vi "XMTmotorSample.vi"() -> ()   [LabVIEW 2018]
uses:
  DLL/XMT_DLL_SER.dll
panel:
  in  "COM":u64=3
  in  "运行停止":bool
  in  "计数清零":bool
  in  "低分辨率":bool
  in  "高分辨率":bool
  in  "MoveX_f 4":dbl=10.0
  in  "设置运行速度":bool
  out "RData 6":sgl
  out "int":i8
  in  "枚举":enum16{"开环O 79", "闭环C 67"}(ring)
  out "返回类型":u8
  out "ReData":u8
  in  "读取下位机单位":bool
  out "数值":i32
  in  "设置下位机单位":bool
  in  "文本下拉列表":u16(ring) items=["0角秒; ", "1毫弧度; ", "2微弧度; ", "3度; ", "4光栅尺一刻度;"]
  out "RData 5":u8
  in  "读取开闭环":bool
  in  "设置开闭环":bool
  in  "读取最大速度":bool
  in  "tmpflagRe":u8=1
  out "RData 4":sgl
  in  "读取位置信息":bool
  in  "MoveX_f 3":dbl
  in  "设置速度":bool
  in  "JOrXFlag":u8
  out "RData 3":sgl
  in  "ReFlag 3":u8
  in  "返回零位置":bool
  out "RData 2":sgl
  in  "ReFlag 2":u8
  in  "MoveX_f 2":dbl=10.0
  in  "位移增量":bool
  out "错误输出":errorcluster
  in  "停止":bool
  out "RData":sgl
  in  "Address":u8=1
  in  "Ch":u8
  in  "ReFlag":u8
  in  "MoveX_f":dbl=24.0
  in  "绝对位置":bool
  # "开环O:79"
  # "闭环C:67"
  # "0角秒 1毫弧度  2微弧度 3度 4光栅尺一刻度"
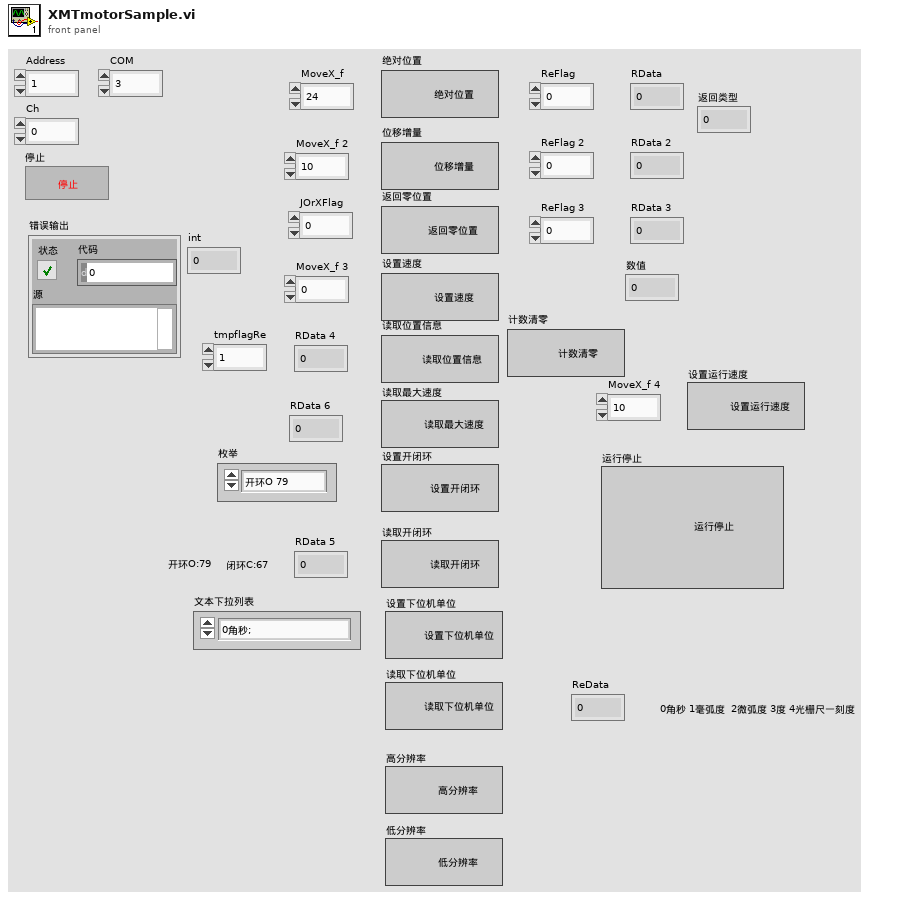
[diagram p1: front panel]
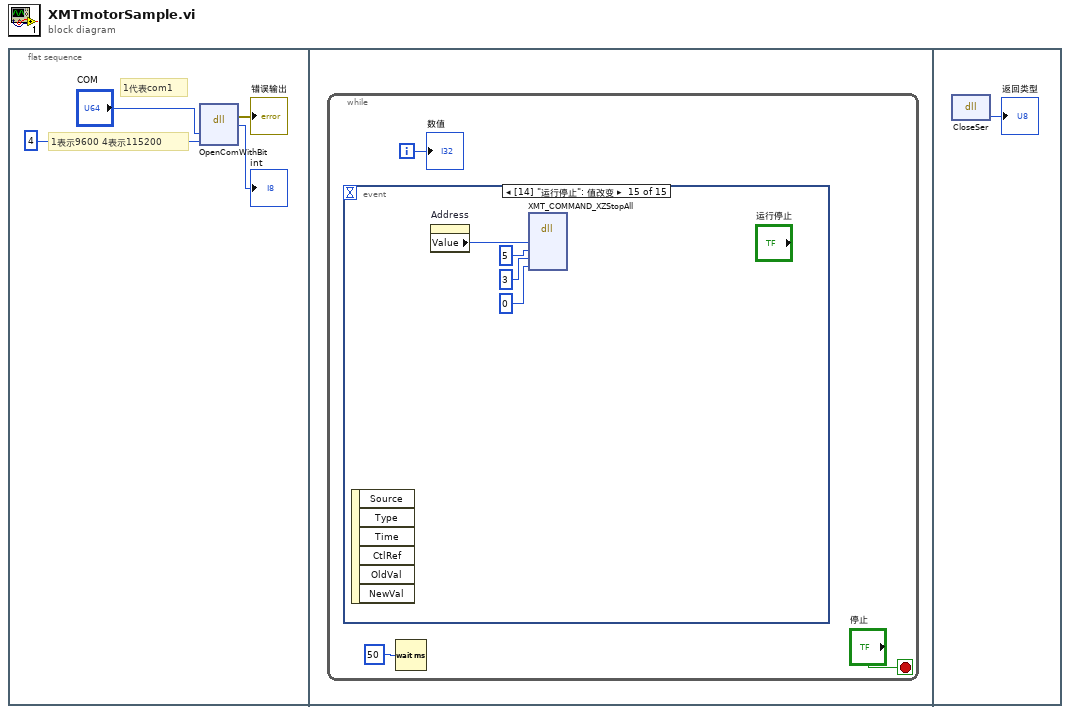
[diagram p0: block diagram]
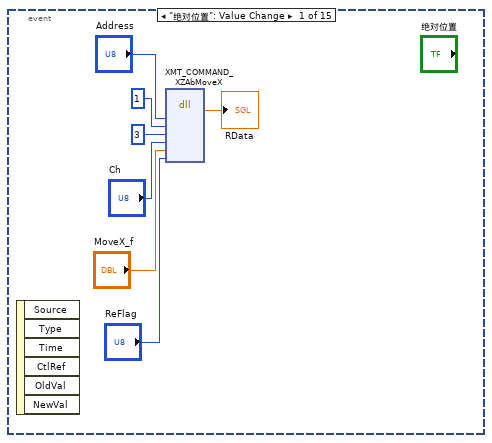
[diagram p2: hidden frame]
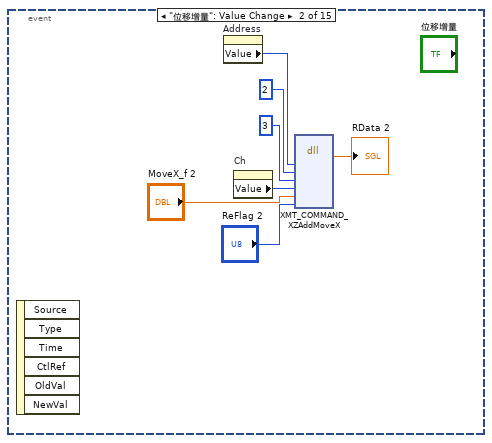
[diagram p3: hidden frame]
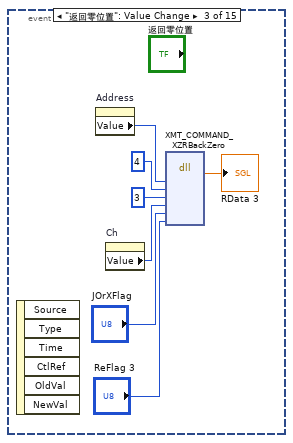
[diagram p4: hidden frame]
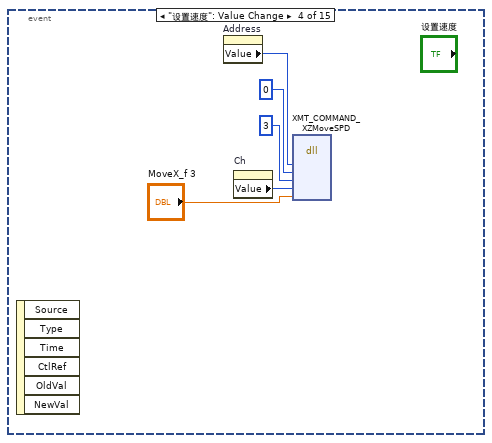
[diagram p5: hidden frame]
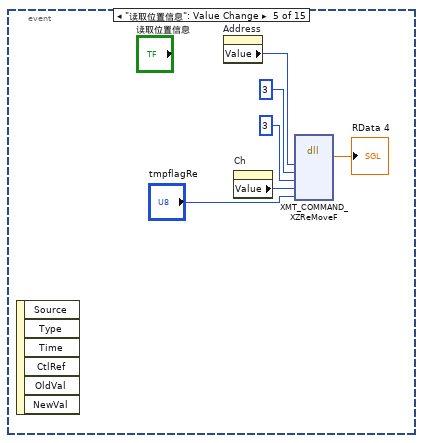
[diagram p6: hidden frame]
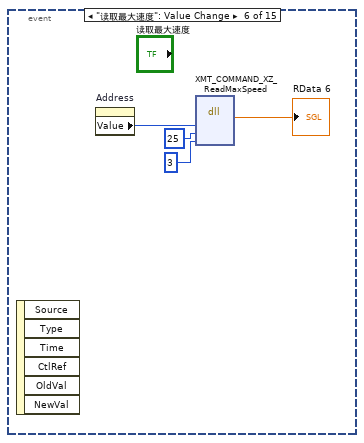
[diagram p7: hidden frame]
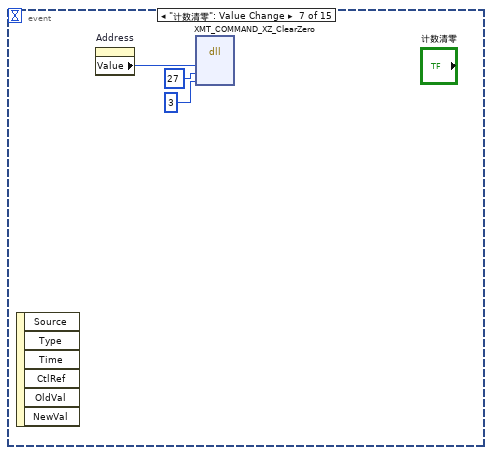
[diagram p8: hidden frame]
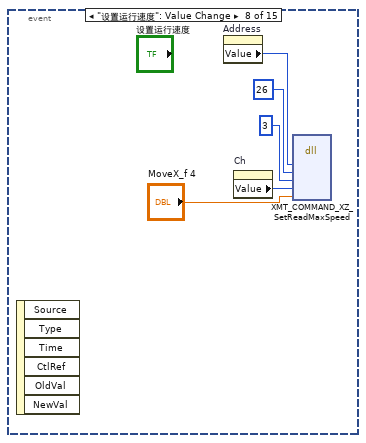
[diagram p9: hidden frame]
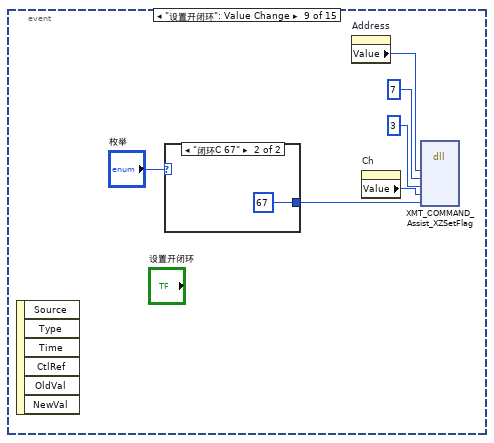
[diagram p10: hidden frame]
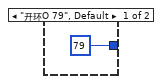
[diagram p11: hidden frame]
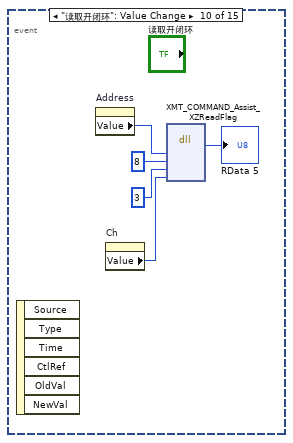
[diagram p12: hidden frame]
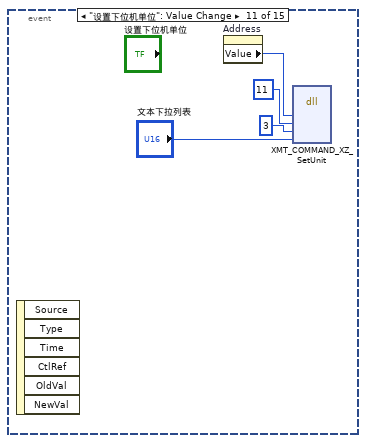
[diagram p13: hidden frame]
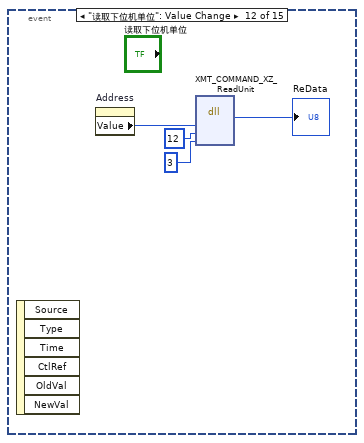
[diagram p14: hidden frame]
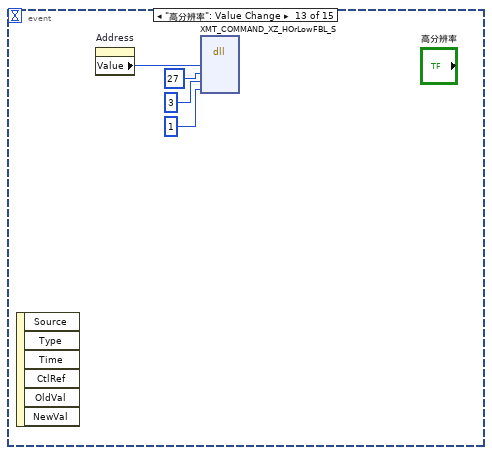
[diagram p15: hidden frame]
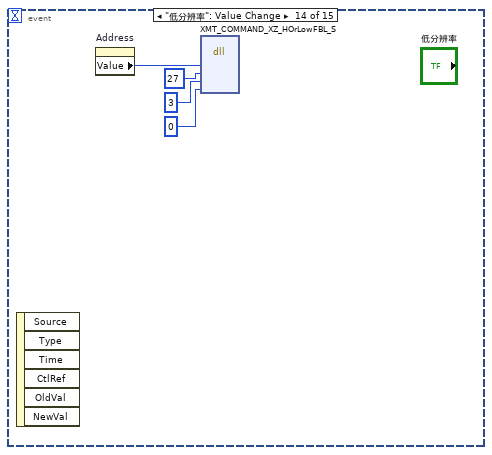
[diagram p16: hidden frame]
diagram:
  n1 = flat-sequence {
    frame #0 {
      # "1表示9600 4表示115200"
      # "1代表com1"
      n2 = dll-call lib="C:/Users/cy3486/OneDrive/Desktop/OPO_control_scripts/SHG_motor_control/DLL/XMT_DLL_SER.dll" fn="OpenComWithBit"("m_com"="COM", "BaudRate"=u8 4) -> (error out=→"错误输出":errorcluster, "int"=→"int":i8)  [unwired: 5 in, 1 out]
    }
    frame #1 {
      n3 = while {
        i -> [w5]
        stop <- "停止" stop-if-true
        n4 = event shown="[14] \"运行停止\": 值改变" {
          selector: _ -> [_ _ _ _ _ _ _ _ _ _ _ _ _ _ _]
          dyn-events: _ -> [_ _ _ _ _ _ _ _ _ _ _ _ _ _ _]
          timeout: _ -> [_ _ _ _ _ _ _ _ _ _ _ _ _ _ _]
          event "绝对位置": Value Change {
            n5 = event-data() -> ()  [unwired: 1 in, 6 out]
            n6 = dll-call lib="C:/Users/cy3486/OneDrive/Desktop/OPO_control_scripts/SHG_motor_control/DLL/XMT_DLL_SER.dll" fn="XMT_COMMAND_XZAbMoveX"("Address"="Address", "Command_B3"=u16 1, "Command_B4"=u16 3 ("Command_B3"), "Ch"="Ch", "MoveX_f"="MoveX_f", "ReFlag"="ReFlag") -> ("RData"=→"RData":sgl)  [unwired: 9 in, 2 out]
          }
          event "位移增量": Value Change {
            n7 = event-data() -> ()  [unwired: 1 in, 6 out]
            n8 = property on="Address" class="DigNum (严格)"() -> ("Value"=w15:u8)  [unwired: 2 in, 2 out]
            n9 = property on="Ch" class="DigNum (严格)"() -> ("Value"=w16:u8)  [unwired: 2 in, 2 out]
            n10 = dll-call lib="C:/Users/cy3486/OneDrive/Desktop/OPO_control_scripts/SHG_motor_control/DLL/XMT_DLL_SER.dll" fn="XMT_COMMAND_XZAddMoveX"("Address"=w15, "Command_B3"=u16 2, "Command_B4"=u16 3 ("Command_B3"), "Ch"=w16, "MoveX_f"="MoveX_f 2", "ReFlag"="ReFlag 2") -> ("RData"=→"RData 2":sgl)  [unwired: 9 in, 2 out]
          }
          event "返回零位置": Value Change {
            n11 = event-data() -> ()  [unwired: 1 in, 6 out]
            n12 = property on="Address" class="DigNum (严格)"() -> ("Value"=w24:u8)  [unwired: 2 in, 2 out]
            n13 = property on="Ch" class="DigNum (严格)"() -> ("Value"=w23:u8)  [unwired: 2 in, 2 out]
            n14 = dll-call lib="C:/Users/cy3486/OneDrive/Desktop/OPO_control_scripts/SHG_motor_control/DLL/XMT_DLL_SER.dll" fn="XMT_COMMAND_XZRBackZero"("Address"=w24, "Command_B3"=u16 4, "Command_B4"=u16 3 ("Command_B3"), "Ch"=w23, "JOrXFlag"="JOrXFlag", "ReFlag"="ReFlag 3") -> ("RData"=→"RData 3":sgl)  [unwired: 9 in, 2 out]
          }
          event "设置速度": Value Change {
            n15 = event-data() -> ()  [unwired: 1 in, 6 out]
            n16 = property on="Address" class="DigNum (严格)"() -> ("Value"=w30:u8)  [unwired: 2 in, 2 out]
            n17 = property on="Ch" class="DigNum (严格)"() -> ("Value"=w31:u8)  [unwired: 2 in, 2 out]
            n18 = dll-call lib="C:/Users/cy3486/OneDrive/Desktop/OPO_control_scripts/SHG_motor_control/DLL/XMT_DLL_SER.dll" fn="XMT_COMMAND_XZMoveSPD"("Address"=w30, "Command_B3"=u16 0, "Command_B4"=u16 3 ("Command_B3"), "Ch"=w31, "MoveX_f"="MoveX_f 3") -> ()  [unwired: 9 in, 2 out]
          }
          event "读取位置信息": Value Change {
            n19 = event-data() -> ()  [unwired: 1 in, 6 out]
            n20 = property on="Address" class="DigNum (严格)"() -> ("Value"=w35:u8)  [unwired: 2 in, 2 out]
            n21 = property on="Ch" class="DigNum (严格)"() -> ("Value"=w36:u8)  [unwired: 2 in, 2 out]
            n22 = dll-call lib="C:/Users/cy3486/OneDrive/Desktop/OPO_control_scripts/SHG_motor_control/DLL/XMT_DLL_SER.dll" fn="XMT_COMMAND_XZReMoveF"("Address"=w35, "Command_B3"=u16 3, "Command_B4"=u16 3 ("Command_B3"), "Ch"=w36, "tmpflagRe"="tmpflagRe") -> ("RData"=→"RData 4":sgl)  [unwired: 8 in, 2 out]
          }
          event "读取最大速度": Value Change {
            n23 = event-data() -> ()  [unwired: 1 in, 6 out]
            n24 = property on="Address" class="DigNum (严格)"() -> ("Value"=w41:u8)  [unwired: 2 in, 2 out]
            n25 = dll-call lib="C:/Users/cy3486/OneDrive/Desktop/OPO_control_scripts/SHG_motor_control/DLL/XMT_DLL_SER.dll" fn="XMT_COMMAND_XZ_ReadMaxSpeed"("Address"=w41, "Command_B3"=u16 25, "Command_B4"=u16 3 ("Command_B3")) -> ("RData"=→"RData 6":sgl)  [unwired: 6 in, 2 out]
          }
          event "计数清零": Value Change {
            n26 = event-data() -> ()  [unwired: 1 in, 6 out]
            n27 = property on="Address" class="DigNum (严格)"() -> ("Value"=w44:u8)  [unwired: 2 in, 2 out]
            n28 = dll-call lib="C:/Users/cy3486/OneDrive/Desktop/OPO_control_scripts/SHG_motor_control/DLL/XMT_DLL_SER.dll" fn="XMT_COMMAND_XZ_ClearZero"("Address"=w44, "Command_B3"=u16 27, "Command_B4"=u16 3 ("Command_B3")) -> ()  [unwired: 7 in, 2 out]
          }
          event "设置运行速度": Value Change {
            n29 = event-data() -> ()  [unwired: 1 in, 6 out]
            n30 = property on="Address" class="DigNum (严格)"() -> ("Value"=w48:u8)  [unwired: 2 in, 2 out]
            n31 = property on="Ch" class="DigNum (严格)"() -> ("Value"=w49:u8)  [unwired: 2 in, 2 out]
            n32 = dll-call lib="C:/Users/cy3486/OneDrive/Desktop/OPO_control_scripts/SHG_motor_control/DLL/XMT_DLL_SER.dll" fn="XMT_COMMAND_XZ_SetReadMaxSpeed"("Address"=w48, "Command_B3"=u16 26, "Command_B4"=u16 3 ("Command_B3"), "Ch"=w49, "MoveX_f"="MoveX_f 4") -> ()  [unwired: 9 in, 2 out]
          }
          event "设置开闭环": Value Change {
            n33 = event-data() -> ()  [unwired: 1 in, 6 out]
            n34 = case shown="\"闭环C 67\"" "枚举" {
              tunnel: [79 67] -> w52
              frame "开环O 79", Default {
              }
              frame "闭环C 67" {
              }
            }
            n35 = property on="Address" class="DigNum (严格)"() -> ("Value"=w54:u8)  [unwired: 2 in, 2 out]
            n36 = property on="Ch" class="DigNum (严格)"() -> ("Value"=w55:u8)  [unwired: 2 in, 2 out]
            n37 = dll-call lib="C:/Users/cy3486/OneDrive/Desktop/OPO_control_scripts/SHG_motor_control/DLL/XMT_DLL_SER.dll" fn="XMT_COMMAND_Assist_XZSetFlag"("Address"=w54, "Command_B3"=u16 7, "Command_B4"=u16 3 ("Command_B3"), "Ch"=w55, "SetFalg"=w52) -> ()  [unwired: 9 in, 2 out]
          }
          event "读取开闭环": Value Change {
            n38 = event-data() -> ()  [unwired: 1 in, 6 out]
            n39 = property on="Address" class="DigNum (严格)"() -> ("Value"=w61:u8)  [unwired: 2 in, 2 out]
            n40 = property on="Ch" class="DigNum (严格)"() -> ("Value"=w62:u8)  [unwired: 2 in, 2 out]
            n41 = dll-call lib="C:/Users/cy3486/OneDrive/Desktop/OPO_control_scripts/SHG_motor_control/DLL/XMT_DLL_SER.dll" fn="XMT_COMMAND_Assist_XZReadFlag"("Address"=w61, "Command_B3"=u16 8, "Command_B4"=u16 3 ("Command_B3"), "Ch"=w62) -> ("RData"=→"RData 5":u8)  [unwired: 7 in, 2 out]
          }
          event "设置下位机单位": Value Change {
            n42 = event-data() -> ()  [unwired: 1 in, 6 out]
            n43 = property on="Address" class="DigNum (严格)"() -> ("Value"=w68:u8)  [unwired: 2 in, 2 out]
            n44 = dll-call lib="C:/Users/cy3486/OneDrive/Desktop/OPO_control_scripts/SHG_motor_control/DLL/XMT_DLL_SER.dll" fn="XMT_COMMAND_XZ_SetUnit"("Address"=w68, "Command_B3"=u16 11, "Command_B4"=u16 3 ("Command_B3"), "UnitFlag"="文本下拉列表") -> ()  [unwired: 8 in, 2 out]
          }
          event "读取下位机单位": Value Change {
            n45 = event-data() -> ()  [unwired: 1 in, 6 out]
            n46 = property on="Address" class="DigNum (严格)"() -> ("Value"=w72:u8)  [unwired: 2 in, 2 out]
            n47 = dll-call lib="C:/Users/cy3486/OneDrive/Desktop/OPO_control_scripts/SHG_motor_control/DLL/XMT_DLL_SER.dll" fn="XMT_COMMAND_XZ_ReadUnit"("address"=w72, "Command_B3"=u16 12, "Command_B4"=u16 3 ("Command_B3")) -> ("ReData"=→"ReData":u8)  [unwired: 6 in, 2 out]
          }
          event "高分辨率": Value Change {
            n48 = event-data() -> ()  [unwired: 1 in, 6 out]
            n49 = property on="Address" class="DigNum (严格)"() -> ("Value"=w74:u8)  [unwired: 2 in, 2 out]
            n50 = dll-call lib="C:/Users/cy3486/OneDrive/Desktop/OPO_control_scripts/SHG_motor_control/DLL/XMT_DLL_SER.dll" fn="XMT_COMMAND_XZ_HOrLowFBL_S"("Address"=w74, "Command_B3"=u16 27, "Command_B4"=u16 3 ("Command_B3"), "HorLowFlag"=u16 1 ("Command_B3")) -> ()  [unwired: 8 in, 2 out]
          }
          event "低分辨率": Value Change {
            n51 = event-data() -> ()  [unwired: 1 in, 6 out]
            n52 = property on="Address" class="DigNum (严格)"() -> ("Value"=w78:u8)  [unwired: 2 in, 2 out]
            n53 = dll-call lib="C:/Users/cy3486/OneDrive/Desktop/OPO_control_scripts/SHG_motor_control/DLL/XMT_DLL_SER.dll" fn="XMT_COMMAND_XZ_HOrLowFBL_S"("Address"=w78, "Command_B3"=u16 27, "Command_B4"=u16 3 ("Command_B3"), "HorLowFlag"=u16 0 ("Command_B3")) -> ()  [unwired: 8 in, 2 out]
          }
          event "运行停止": Value Change {
            n54 = event-data() -> ()  [unwired: 1 in, 6 out]
            n55 = property on="Address" class="DigNum (严格)"() -> ("Value"=w82:u8)  [unwired: 2 in, 2 out]
            n56 = dll-call lib="C:/Users/cy3486/OneDrive/Desktop/OPO_control_scripts/SHG_motor_control/DLL/XMT_DLL_SER.dll" fn="XMT_COMMAND_XZStopAll"("Address"=w82, "Command_B3"=u16 5, "Command_B4"=u16 3 ("Command_B3"), "Channel_Num"=u16 0 ("Command_B3")) -> ()  [unwired: 8 in, 2 out]
          }
        }
        n57 = Wait (ms)(milliseconds to wait=u32 50 ("等待时间（毫秒）")) -> ()  [unwired: 1 out]
        "数值" <- w5
      }
    }
    frame #2 {
      n58 = dll-call lib="C:/Users/cy3486/OneDrive/Desktop/OPO_control_scripts/SHG_motor_control/DLL/XMT_DLL_SER.dll" fn="CloseSer"() -> ("返回类型"=→"返回类型":u8)  [unwired: 3 in, 2 out]
    }
  }
